vi "clib_FGV.vi"(7 "command":T10, 8 "error in (no error)":errorcluster, 9 "Cam Cluster out 2":T1={"incident ANGLE COMPENSATION"=[], "dp/B [MeV/C/B]"=[], "charge compensation"=[], "Momentum [MeV/C]"=[], "energyDependence Input"=[], "pixel angle (y)"=[], "dp [MeV/C/] "=[], "angle 2Dfor spectrumj"=[], "dp [MeV/C] 2D"=[], "charge compensation 2D"=[], "Screen&Camera 2"={"Screen Orientation"="Regular", "Screen angle"="Flat", "Lens"=enum."FL1-f8x08", "Calibration (mm/pix)"=1.0}, "ROI info"={"npix-X"=0, "npix-Y"=0, "Left [pix]"=0.0, "Top [pix]"=0.0}, "Y 2D full angle"=[], "calib pixel"={"y1(pixel)"=[], "y2(pixel)"=[], "dp/B [MeV/C/B] (pixel)"=[], "energyDependence Input(pixel)"=[], "bending angle [deg](pixel)"=[], "total path(pixel)"=[], "pixel angle (y)(pixel)"=[], "energy dependence (pixel)"=[], "charge compensation (pixel)"=[], "Momentum [MeV/C](pixel)"=[], "angular compensation(pixel)"=[]}, "2D"={"dp"=[], "chargeCompensation"=[], "angle"=[], "Momentum"=[]}, "UserROI"={"Width"=0.0, "Hight"=0.0, "OffsetX"=0.0, "OffsetY"=0.0}, "final"={"X"=[], "xi"=[], "delta momentum"=0.0, "Y"=[], "yi"=[], "angle (Y)"=[], "delta angle"=0.0, "scale delta angle"=0.0, "intraX"=0.0, "intraY"=0.0, "mask"=[]}, "B[T]"=0.0, "index"=0.0}, 10 "index":i32, 11 "Clibration":T9={"cam 0"={"incident ANGLE COMPENSATION"=[], "dp/B [MeV/C/B]"=[], "charge compensation"=[], "Momentum [MeV/C]"=[], "energyDependence Input"=[], "pixel angle (y)"=[], "dp [MeV/C/] "=[], "angle 2Dfor spectrumj"=[], "dp [MeV/C] 2D"=[], "charge compensation 2D"=[], "Screen&Camera 2"={"Screen Orientation"="Regular", "Screen angle"="Flat", "Lens"=enum."FL1-f8x08", "Calibration (mm/pix)"=1.0}, "ROI info"={"npix-X"=0, "npix-Y"=0, "Left [pix]"=0.0, "Top [pix]"=0.0}, "Y 2D full angle"=[], "calib pixel"={"y1(pixel)"=[], "y2(pixel)"=[], "dp/B [MeV/C/B] (pixel)"=[], "energyDependence Input(pixel)"=[], "bending angle [deg](pixel)"=[], "total path(pixel)"=[], "pixel angle (y)(pixel)"=[], "energy dependence (pixel)"=[], "charge compensation (pixel)"=[], "Momentum [MeV/C](pixel)"=[], "angular compensation(pixel)"=[]}, "2D"={"dp"=[], "chargeCompensation"=[], "angle"=[], "Momentum"=[]}, "UserROI"={"Width"=0.0, "Hight"=0.0, "OffsetX"=0.0, "OffsetY"=0.0}, "final"={"X"=[], "xi"=[], "delta momentum"=0.0, "Y"=[], "yi"=[], "angle (Y)"=[], "delta angle"=0.0, "scale delta angle"=0.0, "intraX"=0.0, "intraY"=0.0, "mask"=[]}, "B[T]"=0.0, "index"=0.0}, "cam 1"={"incident ANGLE COMPENSATION"=[], "dp/B [MeV/C/B]"=[], "charge compensation"=[], "Momentum [MeV/C]"=[], "energyDependence Input"=[], "pixel angle (y)"=[], "dp [MeV/C/] "=[], "angle 2Dfor spectrumj"=[], "dp [MeV/C] 2D"=[], "charge compensation 2D"=[], "Screen&Camera 2"={"Screen Orientation"="Regular", "Screen angle"="Flat", "Lens"=enum."FL1-f8x08", "Calibration (mm/pix)"=1.0}, "ROI info"={"npix-X"=0, "npix-Y"=0, "Left [pix]"=0.0, "Top [pix]"=0.0}, "Y 2D full angle"=[], "calib pixel"={"y1(pixel)"=[], "y2(pixel)"=[], "dp/B [MeV/C/B] (pixel)"=[], "energyDependence Input(pixel)"=[], "bending angle [deg](pixel)"=[], "total path(pixel)"=[], "pixel angle (y)(pixel)"=[], "energy dependence (pixel)"=[], "charge compensation (pixel)"=[], "Momentum [MeV/C](pixel)"=[], "angular compensation(pixel)"=[]}, "2D"={"dp"=[], "chargeCompensation"=[], "angle"=[], "Momentum"=[]}, "UserROI"={"Width"=0.0, "Hight"=0.0, "OffsetX"=0.0, "OffsetY"=0.0}, "final"={"X"=[], "xi"=[], "delta momentum"=0.0, "Y"=[], "yi"=[], "angle (Y)"=[], "delta angle"=0.0, "scale delta angle"=0.0, "intraX"=0.0, "intraY"=0.0, "mask"=[]}, "B[T]"=0.0, "index"=0.0}, "cam 2"={"incident ANGLE COMPENSATION"=[], "dp/B [MeV/C/B]"=[], "charge compensation"=[], "Momentum [MeV/C]"=[], "energyDependence Input"=[], "pixel angle (y)"=[], "dp [MeV/C/] "=[], "angle 2Dfor spectrumj"=[], "dp [MeV/C] 2D"=[], "charge compensation 2D"=[], "Screen&Camera 2"={"Screen Orientation"="Regular", "Screen angle"="Flat", "Lens"=enum."FL1-f8x08", "Calibration (mm/pix)"=1.0}, "ROI info"={"npix-X"=0, "npix-Y"=0, "Left [pix]"=0.0, "Top [pix]"=0.0}, "Y 2D full angle"=[], "calib pixel"={"y1(pixel)"=[], "y2(pixel)"=[], "dp/B [MeV/C/B] (pixel)"=[], "energyDependence Input(pixel)"=[], "bending angle [deg](pixel)"=[], "total path(pixel)"=[], "pixel angle (y)(pixel)"=[], "energy dependence (pixel)"=[], "charge compensation (pixel)"=[], "Momentum [MeV/C](pixel)"=[], "angular compensation(pixel)"=[]}, "2D"={"dp"=[], "chargeCompensation"=[], "angle"=[], "Momentum"=[]}, "UserROI"={"Width"=0.0, "Hight"=0.0, "OffsetX"=0.0, "OffsetY"=0.0}, "final"={"X"=[], "xi"=[], "delta momentum"=0.0, "Y"=[], "yi"=[], "angle (Y)"=[], "delta angle"=0.0, "scale delta angle"=0.0, "intraX"=0.0, "intraY"=0.0, "mask"=[]}, "B[T]"=0.0, "index"=0.0}, "cam 3"={"incident ANGLE COMPENSATION"=[], "dp/B [MeV/C/B]"=[], "charge compensation"=[], "Momentum [MeV/C]"=[], "energyDependence Input"=[], "pixel angle (y)"=[], "dp [MeV/C/] "=[], "angle 2Dfor spectrumj"=[], "dp [MeV/C] 2D"=[], "charge compensation 2D"=[], "Screen&Camera 2"={"Screen Orientation"="Regular", "Screen angle"="Flat", "Lens"=enum."FL1-f8x08", "Calibration (mm/pix)"=1.0}, "ROI info"={"npix-X"=0, "npix-Y"=0, "Left [pix]"=0.0, "Top [pix]"=0.0}, "Y 2D full angle"=[], "calib pixel"={"y1(pixel)"=[], "y2(pixel)"=[], "dp/B [MeV/C/B] (pixel)"=[], "energyDependence Input(pixel)"=[], "bending angle [deg](pixel)"=[], "total path(pixel)"=[], "pixel angle (y)(pixel)"=[], "energy dependence (pixel)"=[], "charge compensation (pixel)"=[], "Momentum [MeV/C](pixel)"=[], "angular compensation(pixel)"=[]}, "2D"={"dp"=[], "chargeCompensation"=[], "angle"=[], "Momentum"=[]}, "UserROI"={"Width"=0.0, "Hight"=0.0, "OffsetX"=0.0, "OffsetY"=0.0}, "final"={"X"=[], "xi"=[], "delta momentum"=0.0, "Y"=[], "yi"=[], "angle (Y)"=[], "delta angle"=0.0, "scale delta angle"=0.0, "intraX"=0.0, "intraY"=0.0, "mask"=[]}, "B[T]"=0.0, "index"=0.0}}) -> (0 "error out":errorcluster, 3 "Clibration 2":T9={"cam 0"={"incident ANGLE COMPENSATION"=[], "dp/B [MeV/C/B]"=[], "charge compensation"=[], "Momentum [MeV/C]"=[], "energyDependence Input"=[], "pixel angle (y)"=[], "dp [MeV/C/] "=[], "angle 2Dfor spectrumj"=[], "dp [MeV/C] 2D"=[], "charge compensation 2D"=[], "Screen&Camera 2"={"Screen Orientation"="Regular", "Screen angle"="Flat", "Lens"=enum."FL1-f8x08", "Calibration (mm/pix)"=1.0}, "ROI info"={"npix-X"=0, "npix-Y"=0, "Left [pix]"=0.0, "Top [pix]"=0.0}, "Y 2D full angle"=[], "calib pixel"={"y1(pixel)"=[], "y2(pixel)"=[], "dp/B [MeV/C/B] (pixel)"=[], "energyDependence Input(pixel)"=[], "bending angle [deg](pixel)"=[], "total path(pixel)"=[], "pixel angle (y)(pixel)"=[], "energy dependence (pixel)"=[], "charge compensation (pixel)"=[], "Momentum [MeV/C](pixel)"=[], "angular compensation(pixel)"=[]}, "2D"={"dp"=[], "chargeCompensation"=[], "angle"=[], "Momentum"=[]}, "UserROI"={"Width"=0.0, "Hight"=0.0, "OffsetX"=0.0, "OffsetY"=0.0}, "final"={"X"=[], "xi"=[], "delta momentum"=0.0, "Y"=[], "yi"=[], "angle (Y)"=[], "delta angle"=0.0, "scale delta angle"=0.0, "intraX"=0.0, "intraY"=0.0, "mask"=[]}, "B[T]"=0.0, "index"=0.0}, "cam 1"={"incident ANGLE COMPENSATION"=[], "dp/B [MeV/C/B]"=[], "charge compensation"=[], "Momentum [MeV/C]"=[], "energyDependence Input"=[], "pixel angle (y)"=[], "dp [MeV/C/] "=[], "angle 2Dfor spectrumj"=[], "dp [MeV/C] 2D"=[], "charge compensation 2D"=[], "Screen&Camera 2"={"Screen Orientation"="Regular", "Screen angle"="Flat", "Lens"=enum."FL1-f8x08", "Calibration (mm/pix)"=1.0}, "ROI info"={"npix-X"=0, "npix-Y"=0, "Left [pix]"=0.0, "Top [pix]"=0.0}, "Y 2D full angle"=[], "calib pixel"={"y1(pixel)"=[], "y2(pixel)"=[], "dp/B [MeV/C/B] (pixel)"=[], "energyDependence Input(pixel)"=[], "bending angle [deg](pixel)"=[], "total path(pixel)"=[], "pixel angle (y)(pixel)"=[], "energy dependence (pixel)"=[], "charge compensation (pixel)"=[], "Momentum [MeV/C](pixel)"=[], "angular compensation(pixel)"=[]}, "2D"={"dp"=[], "chargeCompensation"=[], "angle"=[], "Momentum"=[]}, "UserROI"={"Width"=0.0, "Hight"=0.0, "OffsetX"=0.0, "OffsetY"=0.0}, "final"={"X"=[], "xi"=[], "delta momentum"=0.0, "Y"=[], "yi"=[], "angle (Y)"=[], "delta angle"=0.0, "scale delta angle"=0.0, "intraX"=0.0, "intraY"=0.0, "mask"=[]}, "B[T]"=0.0, "index"=0.0}, "cam 2"={"incident ANGLE COMPENSATION"=[], "dp/B [MeV/C/B]"=[], "charge compensation"=[], "Momentum [MeV/C]"=[], "energyDependence Input"=[], "pixel angle (y)"=[], "dp [MeV/C/] "=[], "angle 2Dfor spectrumj"=[], "dp [MeV/C] 2D"=[], "charge compensation 2D"=[], "Screen&Camera 2"={"Screen Orientation"="Regular", "Screen angle"="Flat", "Lens"=enum."FL1-f8x08", "Calibration (mm/pix)"=1.0}, "ROI info"={"npix-X"=0, "npix-Y"=0, "Left [pix]"=0.0, "Top [pix]"=0.0}, "Y 2D full angle"=[], "calib pixel"={"y1(pixel)"=[], "y2(pixel)"=[], "dp/B [MeV/C/B] (pixel)"=[], "energyDependence Input(pixel)"=[], "bending angle [deg](pixel)"=[], "total path(pixel)"=[], "pixel angle (y)(pixel)"=[], "energy dependence (pixel)"=[], "charge compensation (pixel)"=[], "Momentum [MeV/C](pixel)"=[], "angular compensation(pixel)"=[]}, "2D"={"dp"=[], "chargeCompensation"=[], "angle"=[], "Momentum"=[]}, "UserROI"={"Width"=0.0, "Hight"=0.0, "OffsetX"=0.0, "OffsetY"=0.0}, "final"={"X"=[], "xi"=[], "delta momentum"=0.0, "Y"=[], "yi"=[], "angle (Y)"=[], "delta angle"=0.0, "scale delta angle"=0.0, "intraX"=0.0, "intraY"=0.0, "mask"=[]}, "B[T]"=0.0, "index"=0.0}, "cam 3"={"incident ANGLE COMPENSATION"=[], "dp/B [MeV/C/B]"=[], "charge compensation"=[], "Momentum [MeV/C]"=[], "energyDependence Input"=[], "pixel angle (y)"=[], "dp [MeV/C/] "=[], "angle 2Dfor spectrumj"=[], "dp [MeV/C] 2D"=[], "charge compensation 2D"=[], "Screen&Camera 2"={"Screen Orientation"="Regular", "Screen angle"="Flat", "Lens"=enum."FL1-f8x08", "Calibration (mm/pix)"=1.0}, "ROI info"={"npix-X"=0, "npix-Y"=0, "Left [pix]"=0.0, "Top [pix]"=0.0}, "Y 2D full angle"=[], "calib pixel"={"y1(pixel)"=[], "y2(pixel)"=[], "dp/B [MeV/C/B] (pixel)"=[], "energyDependence Input(pixel)"=[], "bending angle [deg](pixel)"=[], "total path(pixel)"=[], "pixel angle (y)(pixel)"=[], "energy dependence (pixel)"=[], "charge compensation (pixel)"=[], "Momentum [MeV/C](pixel)"=[], "angular compensation(pixel)"=[]}, "2D"={"dp"=[], "chargeCompensation"=[], "angle"=[], "Momentum"=[]}, "UserROI"={"Width"=0.0, "Hight"=0.0, "OffsetX"=0.0, "OffsetY"=0.0}, "final"={"X"=[], "xi"=[], "delta momentum"=0.0, "Y"=[], "yi"=[], "angle (Y)"=[], "delta angle"=0.0, "scale delta angle"=0.0, "intraX"=0.0, "intraY"=0.0, "mask"=[]}, "B[T]"=0.0, "index"=0.0}})   [LabVIEW 2013]
uses:
  specClustercommandTypdef.ctl
  Calib_Typdef.ctl
  calib_Sub_Typdef.ctl
  ScreenCam2_TypDEf.ctl
  CamAndObj_TypDEf.ctl
  ROIInfo_TypDef.ctl
  calibPixel.ctl
  2DTypDef.ctl
  CamRoiTypDef.ctl
  finalCalibTypdef.ctl
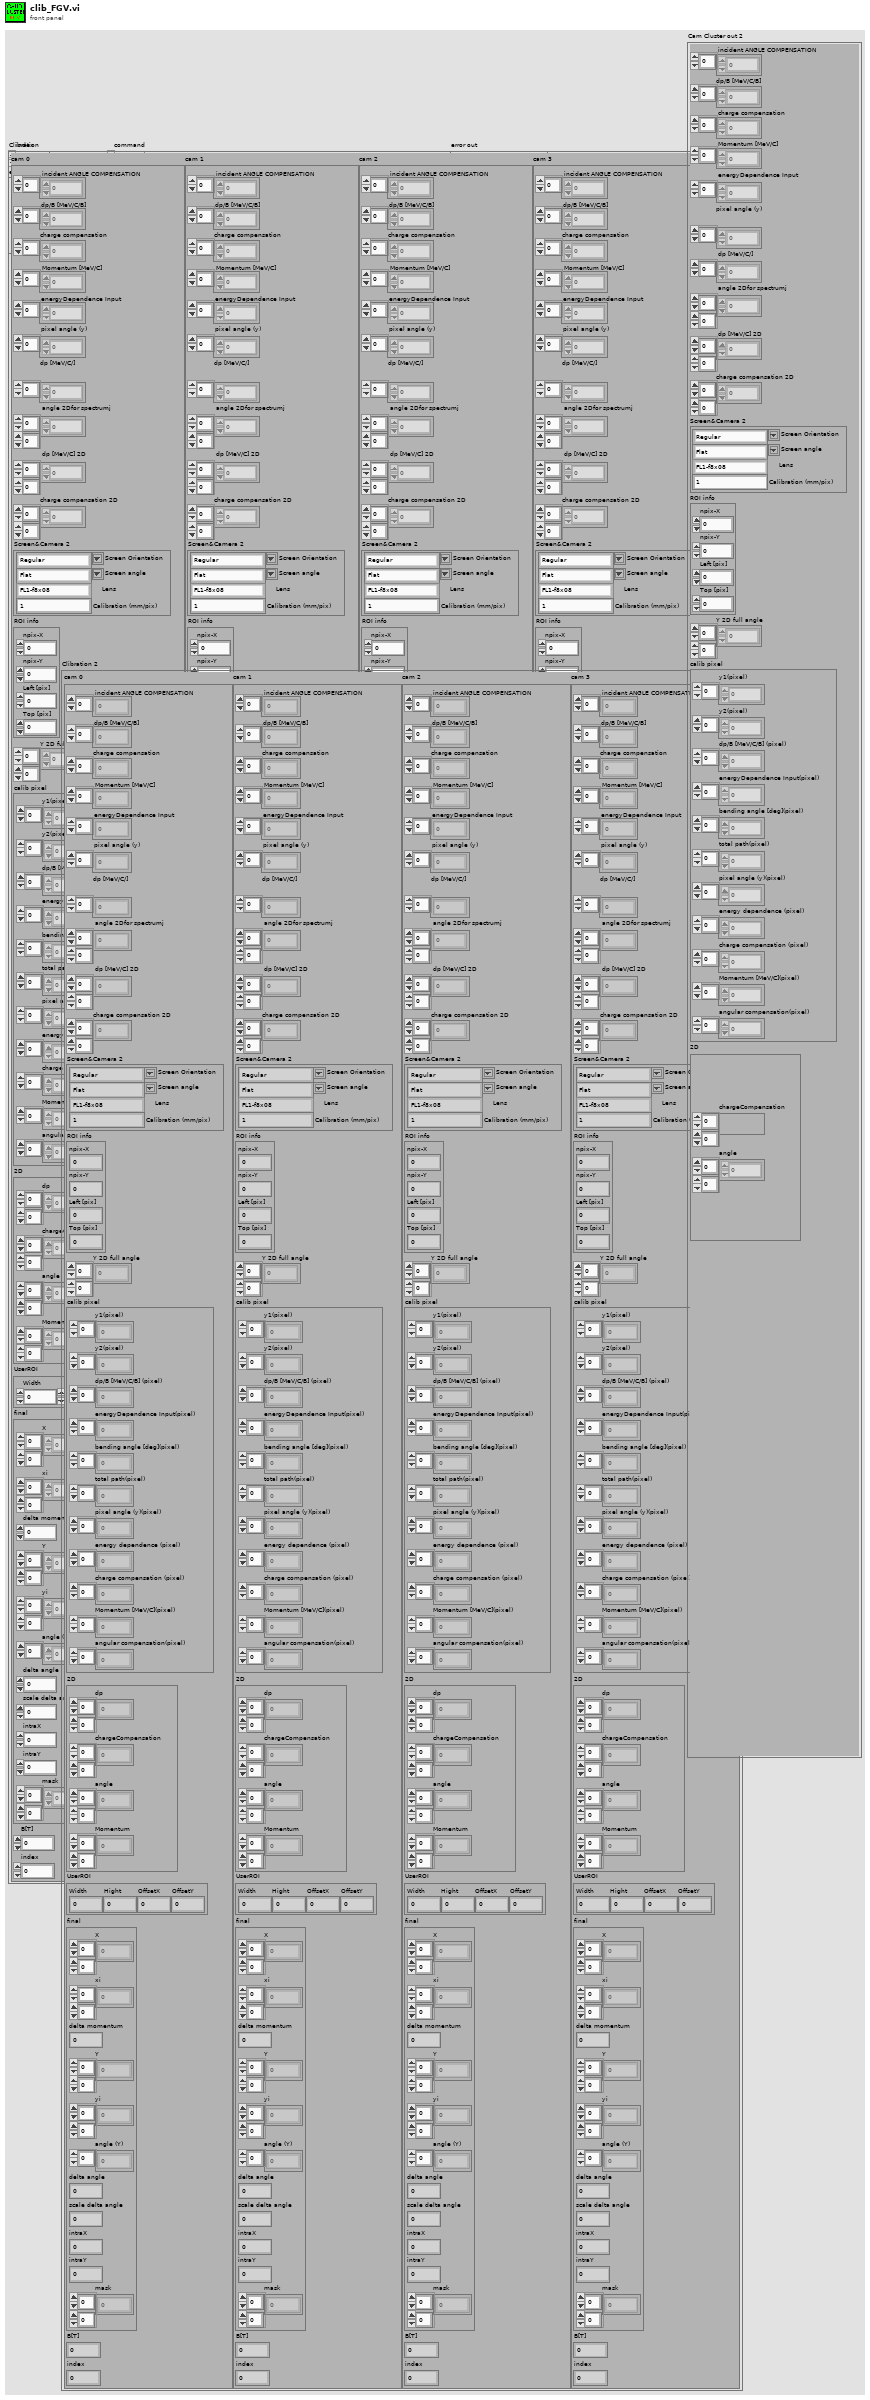
[diagram p1: front panel]
types:
  T1 = typedef "calib_Sub_Typdef.ctl" = cluster{"incident ANGLE COMPENSATION":dbl[], "dp/B [MeV/C/B]":dbl[], "charge compensation":dbl[], "Momentum [MeV/C]":dbl[], "energyDependence Input":dbl[], "pixel angle (y)":dbl[], "dp [MeV/C/] ":dbl[], "angle 2Dfor spectrumj":dbl[][], "dp [MeV/C] 2D":dbl[][], "charge compensation 2D":dbl[][], "Screen&Camera 2":T2, "ROI info":T4, "Y 2D full angle":dbl[][], "calib pixel":T5, "2D":T6, "UserROI":T7, "final":T8, "B[T]":dbl, "index":dbl}
  T2 = typedef "ScreenCam2_TypDEf.ctl" = cluster{"Screen Orientation":string, "Screen angle":string, "Lens":T3, "Calibration (mm/pix)":dbl}
  T3 = typedef "CamAndObj_TypDEf.ctl" = enum16{"FL1-f8x08", "FL1-f8x06", "FL1-f8", "ch300-f50", "FL2G-f8", "FL3M14-f8", "FL3M14-f8x08", "FL3M14-f8x08(2x2)"}
  T4 = typedef "ROIInfo_TypDef.ctl" = cluster{"npix-X":i32, "npix-Y":i32, "Left [pix]":dbl, "Top [pix]":dbl}
  T5 = typedef "calibPixel.ctl" = cluster{"y1(pixel)":dbl[], "y2(pixel)":dbl[], "dp/B [MeV/C/B] (pixel)":dbl[], "energyDependence Input(pixel)":dbl[], "bending angle [deg](pixel)":dbl[], "total path(pixel)":dbl[], "pixel angle (y)(pixel)":dbl[], "energy dependence (pixel)":dbl[], "charge compensation (pixel)":dbl[], "Momentum [MeV/C](pixel)":dbl[], "angular compensation(pixel)":dbl[]}
  T6 = typedef "2DTypDef.ctl" = cluster{"dp":dbl[][], "chargeCompensation":dbl[][], "angle":dbl[][], "Momentum":dbl[][]}
  T7 = typedef "CamRoiTypDef.ctl" = cluster{"Width":dbl, "Hight":dbl, "OffsetX":dbl, "OffsetY":dbl}
  T8 = typedef "finalCalibTypdef.ctl" = cluster{"X":dbl[][], "xi":dbl[][], "delta momentum":dbl, "Y":dbl[][], "yi":dbl[][], "angle (Y)":dbl[], "delta angle":dbl, "scale delta angle":dbl, "intraX":dbl, "intraY":dbl, "mask":dbl[][]}
  T9 = typedef "Calib_Typdef.ctl" = cluster{"cam 0":T1, "cam 1":T1, "cam 2":T1, "cam 3":T1}
  T10 = typedef "specClustercommandTypdef.ctl" = enum16{"init", "addCluster", "read", "clear"}
  T11 = cluster{"Clibration[0]":T1, "Clibration[1]":T1, "Clibration[2]":T1, "Clibration[3]":T1}
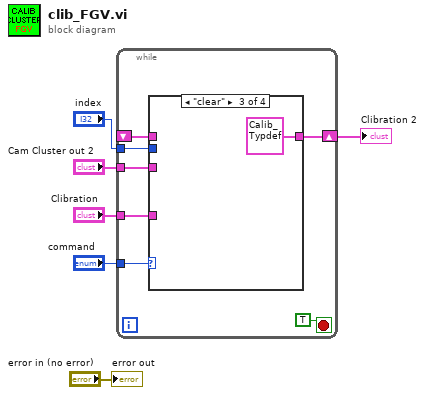
[diagram p0: block diagram]
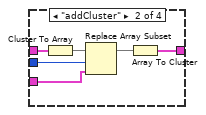
[diagram p3: hidden frame]
diagram:
  n1 = while {
    tunnel: "command" -> [w12]
    shift-right: [w11] -> w2
    shift-left: _ -> [w10]
    tunnel: "Cam Cluster out 2" -> [w8]
    tunnel: "index" -> [w9]
    tunnel: "Clibration" -> [w7]
    stop <- TRUE stop-if-true
    n2 = case shown="\"clear\"" w12 {
      tunnel: [w14 w15 T9 {"cam 0"={"incident ANGLE COMPENSATION"=[], "dp/B [MeV/C/B]"=[], "charge compensation"=[], "Momentum [MeV/C]"=[], "energyDependence Input"=[], "pixel angle (y)"=[], "dp [MeV/C/] "=[], "angle 2Dfor spectrumj"=[], "dp [MeV/C] 2D"=[], "charge compensation 2D"=[], "Screen&Camera 2"={"Screen Orientation"="Regular", "Screen angle"="Flat", "Lens"=enum."FL1-f8x08", "Calibration (mm/pix)"=1.0}, "ROI info"={"npix-X"=0, "npix-Y"=0, "Left [pix]"=0.0, "Top [pix]"=0.0}, "Y 2D full angle"=[], "calib pixel"={"y1(pixel)"=[], "y2(pixel)"=[], "dp/B [MeV/C/B] (pixel)"=[], "energyDependence Input(pixel)"=[], "bending angle [deg](pixel)"=[], "total path(pixel)"=[], "pixel angle (y)(pixel)"=[], "energy dependence (pixel)"=[], "charge compensation (pixel)"=[], "Momentum [MeV/C](pixel)"=[], "angular compensation(pixel)"=[]}, "2D"={"dp"=[], "chargeCompensation"=[], "angle"=[], "Momentum"=[]}, "UserROI"={"Width"=0.0, "Hight"=0.0, "OffsetX"=0.0, "OffsetY"=0.0}, "final"={"X"=[], "xi"=[], "delta momentum"=0.0, "Y"=[], "yi"=[], "angle (Y)"=[], "delta angle"=0.0, "scale delta angle"=0.0, "intraX"=0.0, "intraY"=0.0, "mask"=[]}, "B[T]"=0.0, "index"=0.0}, "cam 1"={"incident ANGLE COMPENSATION"=[], "dp/B [MeV/C/B]"=[], "charge compensation"=[], "Momentum [MeV/C]"=[], "energyDependence Input"=[], "pixel angle (y)"=[], "dp [MeV/C/] "=[], "angle 2Dfor spectrumj"=[], "dp [MeV/C] 2D"=[], "charge compensation 2D"=[], "Screen&Camera 2"={"Screen Orientation"="Regular", "Screen angle"="Flat", "Lens"=enum."FL1-f8x08", "Calibration (mm/pix)"=1.0}, "ROI info"={"npix-X"=0, "npix-Y"=0, "Left [pix]"=0.0, "Top [pix]"=0.0}, "Y 2D full angle"=[], "calib pixel"={"y1(pixel)"=[], "y2(pixel)"=[], "dp/B [MeV/C/B] (pixel)"=[], "energyDependence Input(pixel)"=[], "bending angle [deg](pixel)"=[], "total path(pixel)"=[], "pixel angle (y)(pixel)"=[], "energy dependence (pixel)"=[], "charge compensation (pixel)"=[], "Momentum [MeV/C](pixel)"=[], "angular compensation(pixel)"=[]}, "2D"={"dp"=[], "chargeCompensation"=[], "angle"=[], "Momentum"=[]}, "UserROI"={"Width"=0.0, "Hight"=0.0, "OffsetX"=0.0, "OffsetY"=0.0}, "final"={"X"=[], "xi"=[], "delta momentum"=0.0, "Y"=[], "yi"=[], "angle (Y)"=[], "delta angle"=0.0, "scale delta angle"=0.0, "intraX"=0.0, "intraY"=0.0, "mask"=[]}, "B[T]"=0.0, "index"=0.0}, "cam 2"={"incident ANGLE COMPENSATION"=[], "dp/B [MeV/C/B]"=[], "charge compensation"=[], "Momentum [MeV/C]"=[], "energyDependence Input"=[], "pixel angle (y)"=[], "dp [MeV/C/] "=[], "angle 2Dfor spectrumj"=[], "dp [MeV/C] 2D"=[], "charge compensation 2D"=[], "Screen&Camera 2"={"Screen Orientation"="Regular", "Screen angle"="Flat", "Lens"=enum."FL1-f8x08", "Calibration (mm/pix)"=1.0}, "ROI info"={"npix-X"=0, "npix-Y"=0, "Left [pix]"=0.0, "Top [pix]"=0.0}, "Y 2D full angle"=[], "calib pixel"={"y1(pixel)"=[], "y2(pixel)"=[], "dp/B [MeV/C/B] (pixel)"=[], "energyDependence Input(pixel)"=[], "bending angle [deg](pixel)"=[], "total path(pixel)"=[], "pixel angle (y)(pixel)"=[], "energy dependence (pixel)"=[], "charge compensation (pixel)"=[], "Momentum [MeV/C](pixel)"=[], "angular compensation(pixel)"=[]}, "2D"={"dp"=[], "chargeCompensation"=[], "angle"=[], "Momentum"=[]}, "UserROI"={"Width"=0.0, "Hight"=0.0, "OffsetX"=0.0, "OffsetY"=0.0}, "final"={"X"=[], "xi"=[], "delta momentum"=0.0, "Y"=[], "yi"=[], "angle (Y)"=[], "delta angle"=0.0, "scale delta angle"=0.0, "intraX"=0.0, "intraY"=0.0, "mask"=[]}, "B[T]"=0.0, "index"=0.0}, "cam 3"={"incident ANGLE COMPENSATION"=[], "dp/B [MeV/C/B]"=[], "charge compensation"=[], "Momentum [MeV/C]"=[], "energyDependence Input"=[], "pixel angle (y)"=[], "dp [MeV/C/] "=[], "angle 2Dfor spectrumj"=[], "dp [MeV/C] 2D"=[], "charge compensation 2D"=[], "Screen&Camera 2"={"Screen Orientation"="Regular", "Screen angle"="Flat", "Lens"=enum."FL1-f8x08", "Calibration (mm/pix)"=1.0}, "ROI info"={"npix-X"=0, "npix-Y"=0, "Left [pix]"=0.0, "Top [pix]"=0.0}, "Y 2D full angle"=[], "calib pixel"={"y1(pixel)"=[], "y2(pixel)"=[], "dp/B [MeV/C/B] (pixel)"=[], "energyDependence Input(pixel)"=[], "bending angle [deg](pixel)"=[], "total path(pixel)"=[], "pixel angle (y)(pixel)"=[], "energy dependence (pixel)"=[], "charge compensation (pixel)"=[], "Momentum [MeV/C](pixel)"=[], "angular compensation(pixel)"=[]}, "2D"={"dp"=[], "chargeCompensation"=[], "angle"=[], "Momentum"=[]}, "UserROI"={"Width"=0.0, "Hight"=0.0, "OffsetX"=0.0, "OffsetY"=0.0}, "final"={"X"=[], "xi"=[], "delta momentum"=0.0, "Y"=[], "yi"=[], "angle (Y)"=[], "delta angle"=0.0, "scale delta angle"=0.0, "intraX"=0.0, "intraY"=0.0, "mask"=[]}, "B[T]"=0.0, "index"=0.0}} ("Clibration") w22] -> w11
      tunnel: w10 -> [_ w20 _ w22]
      tunnel: w9 -> [_ w18 _ _]
      tunnel: w8 -> [_ w17 _ _]
      tunnel: w7 -> [w14 _ _ _]
      frame "init", Default {
      }
      frame "addCluster" {
        n3 = Cluster To Array(cluster=w20) -> (array=w19:T1[])
        n4 = Replace Array Subset(array=w19, new element=w17, index=w18) -> (w16:T1[])
        n5 = Array To Cluster(array=w16) -> (cluster=w15:T11)
      }
      frame "clear" {
      }
      frame "read" {
      }
    }
  }
  "Clibration 2" <- w2
  "error out" <- "error in (no error)"
